vi "DVSW Dynamics Viscosity of Saline Water(Kg to m to s).vi"(1 "Salinity":dbl, 2 "Sailne Water Temprature":dbl[unit]) -> (0 "DVSW1.5%":dbl[unit])   [LabVIEW 2018]
panel:
  out "DVSW1%":dbl[unit]
  out "DVPW":dbl[unit]
  out "Saline Water Temprature":dbl[unit](slide) scale=0.0..100.0
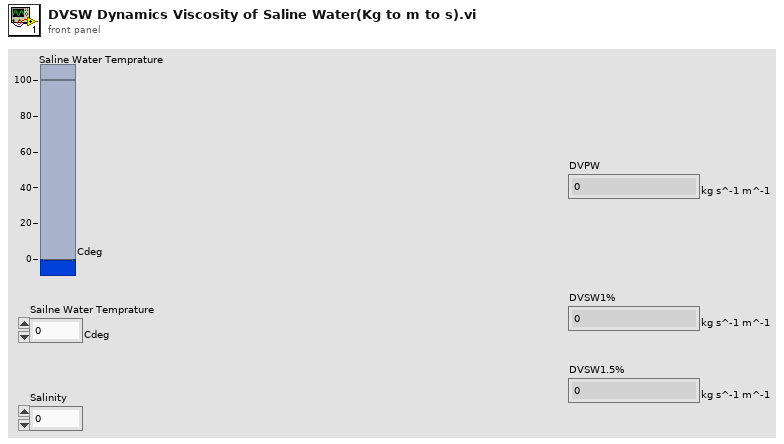
[diagram p1: front panel]
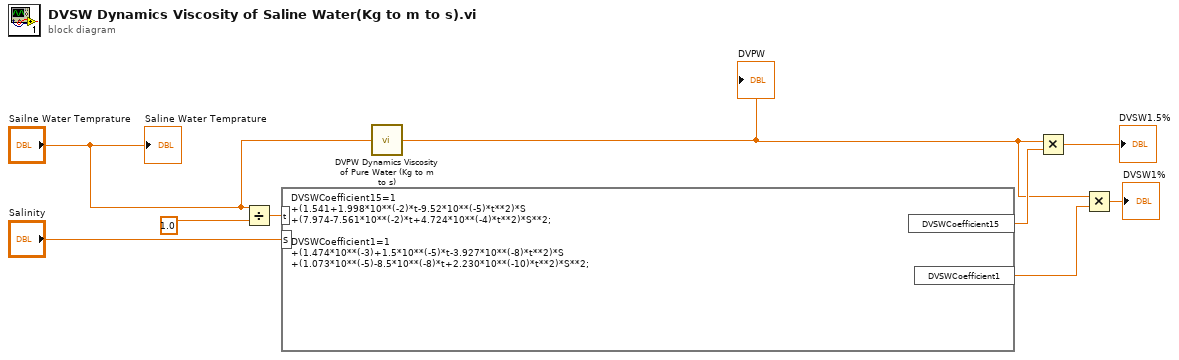
[diagram p0: block diagram]
diagram:
  n1 = Divide(x="Sailne Water Temprature", y=dbl[unit] 1.0) -> (x/y=w9:dbl)
  n2 = formula code="DVSWCoefficient15=1\n+(1.541+1.998*10**(-2)*t-9.52*10**(-5)*t**2)*S\n+(7.974-7.561*10**(-2)*t+4.724*10**(-4)*t**2)*S**2;\n\nDVSWCoefficient1=1\n+(1.474*10**(-3)+1.5*10**(-5)*t-3.927*10**(-8)*t**2)*S\n+(1.073*10**(-5)-8.5*10**(-8)*t+2.230*10**(-10)*t**2)*S**2;"("t"=w9, "S"="Salinity") -> ("DVSWCoefficient15"=w6:dbl, "DVSWCoefficient1"=w2:dbl)
  n3 = call "DVPW Dynamics Viscosity of Pure Water (Kg to m to s).vi"("Pure Water Temprature"="Sailne Water Temprature") -> ("DVPW"=w1:dbl[unit])
  "DVPW" <- w1
  n4 = Multiply(x=w1, y=w6) -> (x*y=→"DVSW1.5%":dbl[unit])
  n5 = Multiply(x=w1, y=w2) -> (x*y=→"DVSW1%":dbl[unit])
  "Saline Water Temprature" <- "Sailne Water Temprature"
